vi "Run All Tests.vi"() -> ()   [LabVIEW 2020]
uses:
  Python Data Tools Tests/Python Data Tools Tests.lvclass
  C:/Program Files/National Instruments/LabVIEW 2020/vi.lib/addons/_JKI Toolkits/VI Tester/TestCase.llb/TestCase.lvclass
  Scan From Python String Tests/Scan From Python String Tests.lvclass
  Python String Parsing Utility Tests/Python String Parsing Utility Tests.lvclass
  <vilib>/addons/_JKI Toolkits/VI Tester/VI Tester API.llb/Run Tests (Test Object Array).vi
  <vilib>/addons/_JKI Toolkits/VI Tester/VI Tester API.llb/VI Tester API.lvlib
  <vilib>/addons/_JKI Toolkits/VI Tester/TestCase.llb/TestCase.lvclass
panel:
  out "successful?":bool
  out "error out":errorcluster
  out "test details":string
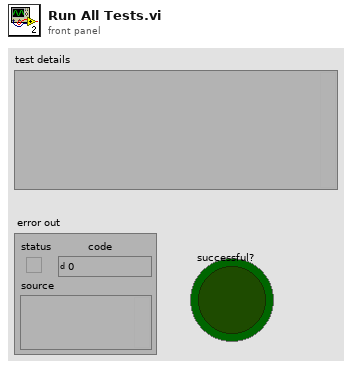
[diagram p1: front panel]
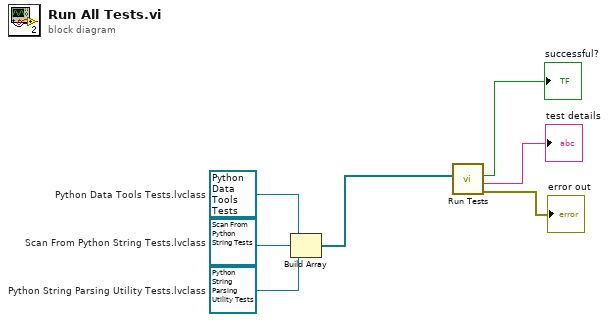
[diagram p0: block diagram]
diagram:
  w5 = refnum<class "Python String Parsing Utility Tests.lvclass"> refnum  # Python String Parsing Utility Tests.lvclass
  w4 = refnum<class "Scan From Python String Tests.lvclass"> refnum  # Scan From Python String Tests.lvclass
  w6 = refnum<class "Python Data Tools Tests.lvclass"> refnum  # Python Data Tools Tests.lvclass
  n1 = Build Array(w6, w4, w5) -> (w3:refnum<class "TestCase.lvclass">[])
  n2 = call-poly <vilib>:"Run Tests.vi"("Tests"=w3) -> ("error out"=→"error out":errorcluster, "test details"=→"test details":string, "successful?"=→"successful?":bool)  [unwired: 8 in]
